vi "Sweeping Turn (Spencer Scott's conflicted copy 2017-03-24).vi"(6 "upper angle limit":dbl, 8 "error in":errorcluster) -> (0 "error out":errorcluster)   [LabVIEW 2016]
uses:
  Robot Global Data.vi
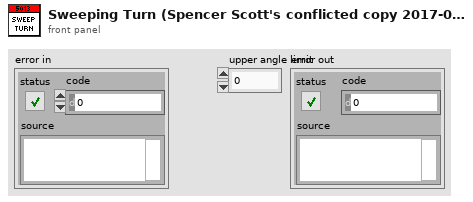
[diagram p1: front panel]
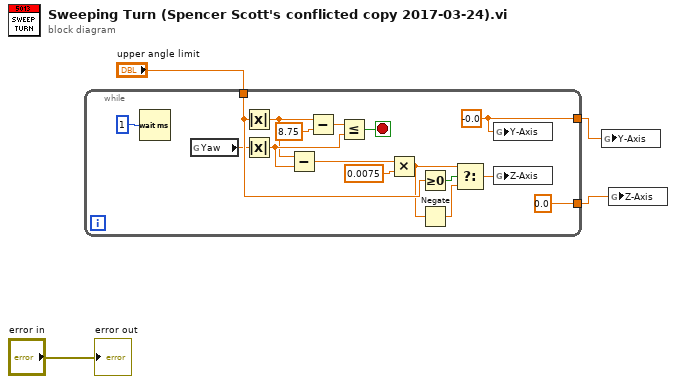
[diagram p0: block diagram]
diagram:
  n1 = while {
    tunnel: "upper angle limit" -> [w17]
    tunnel: [0.0 ("setpoint")] -> w2
    tunnel: [w10] -> w1
    stop <- w18 stop-if-true
    w10 = -0.0 ("Y-Axis")
    n2 = Wait (ms)(milliseconds to wait=u32 1) -> ()  [unwired: 1 out]
    n3 = global read "Robot Global Data.vi" "Yaw"() -> (w11:dbl)
    n4 = Absolute Value(x=w17) -> (abs(x)=w8:dbl)
    n5 = Absolute Value(x=w11) -> (abs(x)=w9:dbl)
    n6 = Subtract(x=w8, y=w9) -> (x-y=w7:dbl)
    n7 = Subtract(x=w8, y=8.75 ("x")) -> (x-y=w13:dbl)
    n8 = Less Or Equal?(x=w13, y=w9) -> (x <= y?=w18:bool)
    n9 = Multiply(x=w7, y=0.0075 ("Y-Axis")) -> (x*y=w5:dbl)
    n10 = Greater Or Equal To 0?(x=w17) -> (x >= 0?=w16:bool)
    n11 = Negate(x=w5) -> (-x=w15:dbl)
    n12 = Select(t=w5, s=w16, f=w15) -> (s? t:f=w14:dbl)
    n13 = global write "Robot Global Data.vi" "Y-Axis"(w10) -> ()
    n14 = global write "Robot Global Data.vi" "Z-Axis"(w14) -> ()
  }
  n15 = global write "Robot Global Data.vi" "Y-Axis"(w1) -> ()
  n16 = global write "Robot Global Data.vi" "Z-Axis"(w2) -> ()
  "error out" <- "error in"
